vi "Geometric CDF.vi"(10 "p":dbl=0.5, 11 "n":dbl=1.0) -> (0 "error":i32, 3 "cdf(n)":dbl=0.75)   [LabVIEW 2017, in "NI_Gmath.lvlib"]
doc: "Computes the discrete cumulative distribution function (CDF), or the probability that the random variate X, where X describes the selected distribution type, takes on a value less than or equal to <B>x</B>. You must manually select the polymorphic instance to use."
uses:
  NI_Gmath.lvlib
panel:
  # "Geometric CDF"
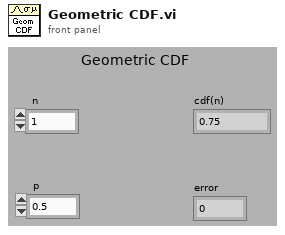
[diagram p1: front panel]
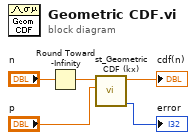
[diagram p0: block diagram]
diagram:
  n1 = Round Toward -Infinity(1:"n") -> (0:w1:dbl)
  n2 = call "st_Geometric CDF (kx).vi"("p"="p", "nx"=w1) -> ("error"=→"error":i32, "cdf(nx)"=→"cdf(n)":dbl)  [unwired: 8 in]
